vi "DHE_GetPrePostNumFrames.vi"() -> (7 "DHE_PreExpose":i32, 9 "DHE_PostExpose":i32)   [LabVIEW 2016]
uses:
  private/vis/DHE_GBLDriverVariables.vi
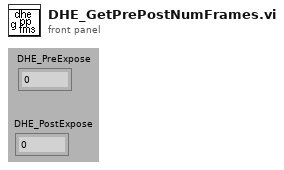
[diagram p1: front panel]
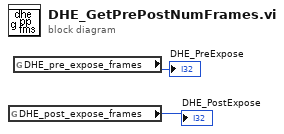
[diagram p0: block diagram]
diagram:
  n1 = global read "DHE_GBLDriverVariables.vi" "DHE_post_expose_frames"() -> (→"DHE_PostExpose":u16)
  n2 = global read "DHE_GBLDriverVariables.vi" "DHE_pre_expose_frames"() -> (→"DHE_PreExpose":u16)
